vi "p1.vi"() -> ()   [LabVIEW 2023, in "d6.lvlib"]
uses:
  d6.lvlib
  <vilib>/Analysis/polynomials.llb/Polynomial Roots (DBL).vi
  <vilib>/regexp/Match Regular Expression.xnode
  AOC/AOC.lvlib
  <vilib>/Analysis/NI_AALPro.lvlib
panel:
  in  "Input":string="Time:        35     69     68     87\nDistance:   213   1168   1086   1248"
  in  "Example":string="Time:      7  15   30\nDistance:  9  40  200"
  in  "Example":bool=TRUE
  out "Answer":i64=1909
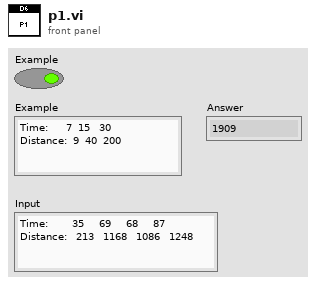
[diagram p1: front panel]
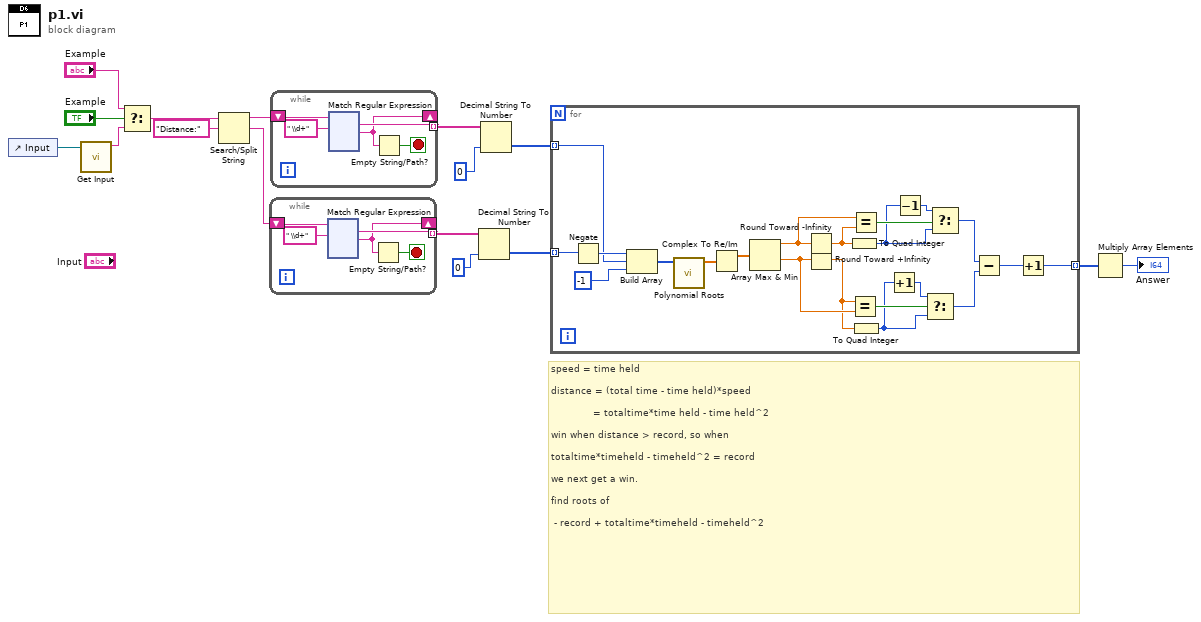
[diagram p0: block diagram]
diagram:
  # "speed = time held\n\ndistance = (total time - time held)*speed\n\n              = totaltime*time held - time held^2\n\nwin when distance > record, so when \n\ntotaltime*timeheld - timeheld^2 = record\n\nwe next get a win.\n\nfind roots of\n\n - record + totaltime*timeheld - timeheld^2"
  n1 = control-ref of="Input"() -> (w1:refnum<vi>)
  n2 = call "Get Input.vi"("Input ref"=w1) -> ("Input"=w16:string)  [unwired: 10 in]
  n3 = Select(t="Example", s="Example", f=w16) -> (s? t:f=w13:string)
  n4 = Search/Split String(string=w13, search string/char (-)="Distance:") -> (substring before match=w11:string, match + rest of string=w10:string)  [unwired: 1 in, 1 out]
  n5 = while {
    tunnel: [w19] -> w8 mode=indexing
    shift-right: [w17] -> _
    shift-left: w10 -> [w21]
    stop <- w18 stop-if-true
    n6 = xnode "Match Regular Expression"("input string"=w21, "regular expression"=" \\d+") -> ("whole match"=w19:string, "after match"=w17:string)  [unwired: 4 in, 3 out]
    n7 = Empty String/Path?(string/path=w17) -> (empty?=w18:bool)
  }
  n8 = while {
    tunnel: [w141] -> w9 mode=indexing
    shift-right: [w139] -> _
    shift-left: w11 -> [w143]
    stop <- w140 stop-if-true
    n9 = xnode "Match Regular Expression"("input string"=w143, "regular expression"=" \\d+") -> ("whole match"=w141:string, "after match"=w139:string)  [unwired: 4 in, 3 out]
    n10 = Empty String/Path?(string/path=w139) -> (empty?=w140:bool)
  }
  n11 = Decimal String To Number(string=w8, default (0L)=i64 0 ("Answer")) -> (number=w4:i64[])  [unwired: 1 in, 1 out]
  n12 = Decimal String To Number(string=w9, default (0L)=i64 0 ("Answer")) -> (number=w5:i64[])  [unwired: 1 in, 1 out]
  n13 = for {
    tunnel: w5 -> [w279] mode=indexing
    tunnel: w4 -> [w281] mode=indexing
    tunnel: [w261] -> w3 mode=indexing
    n14 = Negate(x=w281) -> (-x=w280:i64)
    n15 = Build Array(w280, w279, i64 -1 ("element")) -> (w277:i64[])
    n16 = call-poly <vilib>:"Polynomial Roots.vi"("P(x)"=w277) -> ("Roots"=w276:cdb[])  [unwired: 9 in, 1 out]
    n17 = Complex To Re/Im(x + iy=w276) -> (x=w275:dbl[])  [unwired: 1 out]
    n18 = Array Max & Min(array=w275) -> (max value=w273:dbl, min value=w274:dbl)  [unwired: 2 out]
    n19 = Round Toward -Infinity(1:w273) -> (0:w268:dbl)
    n20 = Round Toward +Infinity(x=w274) -> (ceil(x): smallest int >= x=w266:dbl)
    n21 = To Quad Integer(1:w268) -> (0:w267:i64)
    n22 = Equal?(x=w266, y=w274) -> (x = y?=w272:bool)
    n23 = Equal?(x=w273, y=w268) -> (x = y?=w270:bool)
    n24 = To Quad Integer(1:w266) -> (0:w265:i64)
    n25 = Increment(x=w265) -> (x+1=w271:i64)
    n26 = Decrement(x=w267) -> (x-1=w269:i64)
    n27 = Select(t=w271, s=w272, f=w265) -> (s? t:f=w263:i64)
    n28 = Select(t=w269, s=w270, f=w267) -> (s? t:f=w264:i64)
    n29 = Subtract(x=w264, y=w263) -> (x-y=w262:i64)
    n30 = Increment(x=w262) -> (x+1=w261:i64)
  }
  n31 = Multiply Array Elements(1:w3) -> (0:→"Answer":i64)
